vi "Pressure write test.vi"() -> ()   [LabVIEW 2016]
uses:
  <vilib>/express/express signal manip/GetorSetDDTAttributes/Shared VIs/TimeType.ctl
  <vilib>/express/express signal manip/GetorSetDDTAttributes/Shared VIs/TimeMode Enum to Boolean.vi
  <vilib>/express/express shared/transition.llb/Dynamic To Waveform Array.vi
  <vilib>/express/express signal manip/GetorSetDDTAttributes/Set DDT Attributes/SetT0.vi
  <vilib>/express/express shared/transition.llb/Waveform Array To Dynamic.vi
  <vilib>/express/express signal manip/GetorSetDDTAttributes/Set DDT Attributes/Set DDT Properties.xnode
  <vilib>/express/express signal manip/GetorSetDDTAttributes/Shared VIs/GetSetShared.lvlib
panel:
  in  "Combo Box":string(combo)
  in  "Stop Button":bool
  out "Manifold Pressure":dbl[unit]
  out "Tube Pressure":dbl[unit]
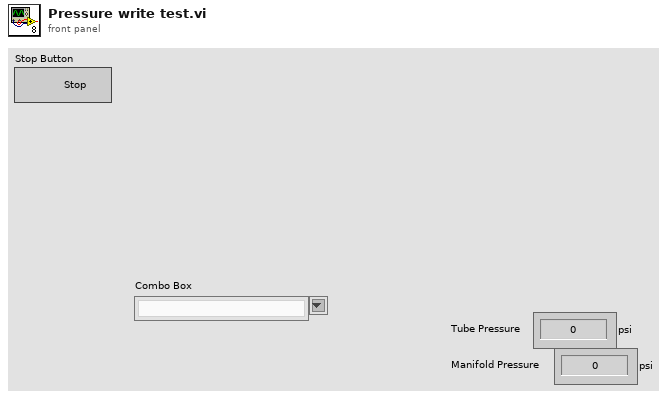
[diagram p1: front panel]
types:
  T1 = typedef "GetSetShared.lvlib/TimeType.ctl" = enum16{"Absolute", "Relative"}
  T2 = cluster{"Time":timestamp, "Tube reading":dbl, "Manifold reading":dbl}
  T3 = cluster{"Manifold slope":dbl, "Manifold intercept":dbl, "Tube slope":dbl, "Tube intercept":dbl}
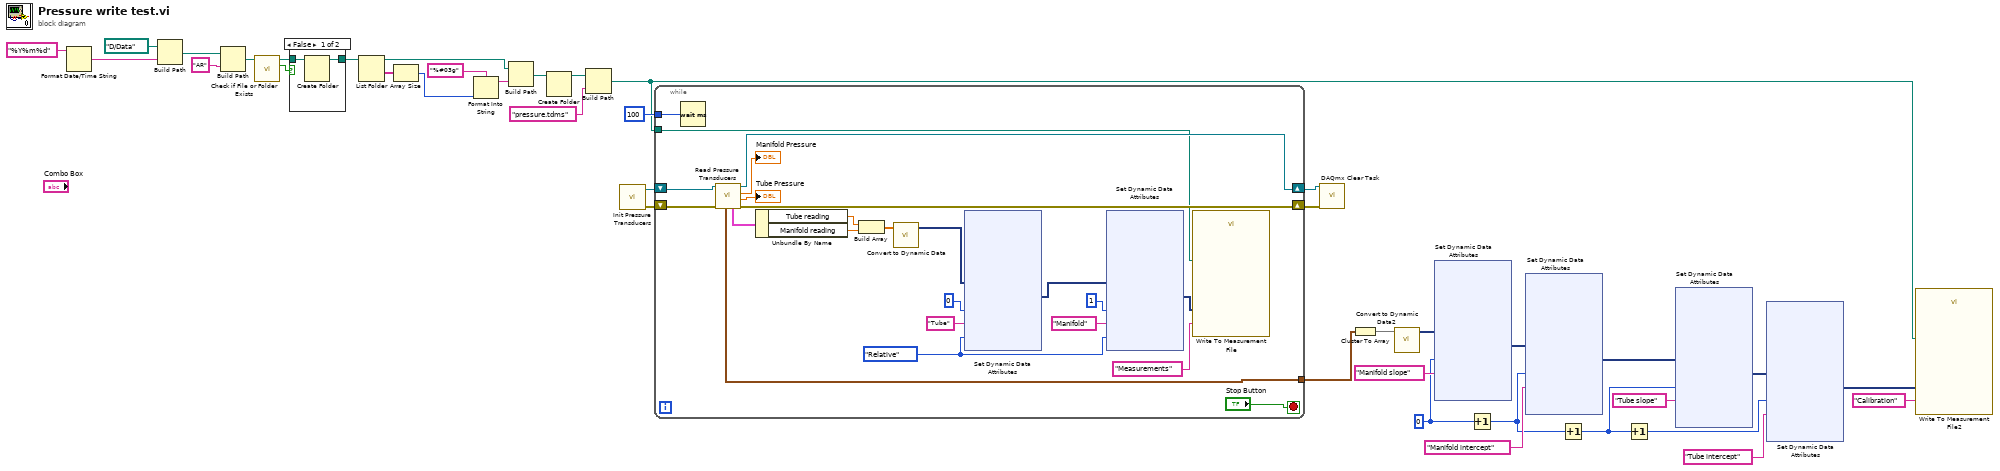
[diagram p0: block diagram]
diagram:
  w23 = 0 ("Signal Index")
  n1 = Format Date/Time String(time format string (%c)="%Y%m%d") -> (date/time string=w16:string)  [unwired: 2 in]
  n2 = Build Path(base path=path "D:/Data", name or relative path=w16) -> (appended path=w15:path)
  n3 = Build Path(base path=w15, name or relative path="AR") -> (appended path=w13:path)
  n4 = call <vilib>:"Check if File or Folder Exists.vi"("path"=w13) -> ("file or folder exists?"=w12:bool, "dup path"=w11:path)  [unwired: 8 in, 1 out]
  n5 = case shown="False" w12 {
    tunnel: w11 -> [w41 w42]
    tunnel: [w40 w42] -> w10
    frame False {
      n6 = Create Folder(path (use dialog)=w41) -> (created path=w40:path)  [unwired: 2 in, 2 out]
    }
    frame True {
    }
  }
  n7 = List Folder(path=w10) -> (path out=w7:path, folder names=w9:string[])  [unwired: 3 in, 2 out]
  n8 = Array Size(array=w9) -> (size(s)=w1:i32)
  n9 = Format Into String(format string="%#03g", w1) -> (resulting string=w6:string)  [unwired: 2 in, 1 out]
  n10 = Build Path(base path=w7, name or relative path=w6) -> (appended path=w5:path)
  n11 = Create Folder(path (use dialog)=w5) -> (created path=w4:path)  [unwired: 2 in, 2 out]
  n12 = Build Path(base path=w4, name or relative path="pressure.tdms") -> (appended path=w2:path)
  n13 = call "Init Pressure Transducers.vi"() -> ("Error Out"=w38:errorcluster, "task out"=w39:refnum<k21>)  [unwired: 1 in]
  n14 = while {
    shift-right: [w61] -> w37
    shift-left: w39 -> [w65]
    shift-right: [w60] -> w36
    shift-left: w38 -> [w64]
    tunnel: u32 100 ("milliseconds to wait") -> [w58]
    tunnel: [w45] -> w34
    tunnel: w2 -> [w43]
    stop <- "Stop Button" stop-if-true
    w46 = TimeType."Relative" ("Time Mode")
    n15 = Wait (ms)(milliseconds to wait=w58) -> ()  [unwired: 1 out]
    n16 = call "Read Pressure Transducers.vi"("Error In"=w64, "task in"=w65) -> ("Error Out"=w60:errorcluster, "Tube Pressure"=→"Tube Pressure":dbl[unit], "Manifold Pressure"=→"Manifold Pressure":dbl[unit], "task out"=w61:refnum<k21>, "Readings"=w59:T2, "Calibration coefficients"=w45:T3)  [unwired: 4 in]
    n17 = Unbundle By Name(w59) -> ("Tube reading"=w50:dbl, "Manifold reading"=w49:dbl)
    n18 = Build Array(w50, w49) -> (w48:dbl[])
    n19 = call "Convert to Dynamic Data"("Array"=w48) -> ("Dynamic Data Type"=w57:dynamicdata)  [unwired: 3 in]
    n20 = xnode "Set Dynamic Data Attributes"("Signals In"=w57, "Signal Index"=0, "Signal Name"="Tube", "Time Mode"=w46) -> ("Signals Out"=w54:dynamicdata)  [unwired: 1 in, 1 out]
    n21 = xnode "Set Dynamic Data Attributes"("Signals In"=w54, "Signal Index"=1, "Signal Name"="Manifold", "Time Mode"=w46) -> ("Signals Out"=w51:dynamicdata)  [unwired: 1 in, 1 out]
    n22 = call "Write To Measurement File"("Signals"=w51, "Filename"=w43, "Comment"="Measurements") -> ()  [unwired: 14 in, 3 out]
  }
  n23 = call <vilib>:"DAQmx Clear Task.vi"("task in"=w37, "error in"=w36) -> ()  [unwired: 13 in, 1 out]
  n24 = Cluster To Array(cluster=w34) -> (array=w33:dbl[])
  n25 = call "Convert to Dynamic Data2"("Array"=w33) -> ("Dynamic Data Type"=w32:dynamicdata)  [unwired: 3 in]
  n26 = xnode "Set Dynamic Data Attributes"("Signals In"=w32, "Signal Index"=w23, "Signal Name"="Manifold slope") -> ("Signals Out"=w31:dynamicdata)  [unwired: 2 in, 1 out]
  n27 = Increment(x=w23) -> (x+1=w22:i32)
  n28 = xnode "Set Dynamic Data Attributes"("Signals In"=w31, "Signal Index"=w22, "Signal Name"="Manifold intercept") -> ("Signals Out"=w30:dynamicdata)  [unwired: 2 in, 1 out]
  n29 = Increment(x=w22) -> (x+1=w21:i32)
  n30 = Increment(x=w21) -> (x+1=w20:i32)
  n31 = xnode "Set Dynamic Data Attributes"("Signals In"=w30, "Signal Index"=w21, "Signal Name"="Tube slope") -> ("Signals Out"=w29:dynamicdata)  [unwired: 2 in, 1 out]
  n32 = xnode "Set Dynamic Data Attributes"("Signals In"=w29, "Signal Index"=w20, "Signal Name"="Tube intercept") -> ("Signals Out"=w28:dynamicdata)  [unwired: 2 in, 1 out]
  n33 = call "Write To Measurement File2"("Signals"=w28, "Filename"=w2, "Comment"="Calibration") -> ()  [unwired: 14 in, 3 out]
